vi "SLL DE AO Continous Engine.vi"(8 "error in (no error)":errorcluster) -> (0 "error out":errorcluster)   [LabVIEW 2013]
doc: "Copyright © 2005, Soliton Technologies.\nAll rights reserved."
uses:
  Controls/SLL DE DAQ Engine Options.ctl
  Controls/SLL DE AO Command LV2Global Options.ctl
  Controls/SLL DE AO Response LV2Global Options.ctl
  Controls/SLL DE AO Global Options.ctl
  Controls/SLL DE AO Circular Buffer Options.ctl
  Controls/SLL DE AO Min Max Range Checking Options.ctl
  Controls/SLL DE DAQ Global Options.ctl
  Controls/SLL DE DAQ Global Elements.ctl
  Controls/SLL DE DAQ Engine Channel Types.ctl
  Controls/SLL DE DAQ Parameters LV2Global Options.ctl
  Controls/SLL DE AO Safe Value Global Options.ctl
  <vilib>/DAQmx/configure/timing.llb/DAQmx Timing (Sample Clock).vi
  <vilib>/DAQmx/write.llb/DAQmx Write (Analog DBL 1Chan 1Samp).vi
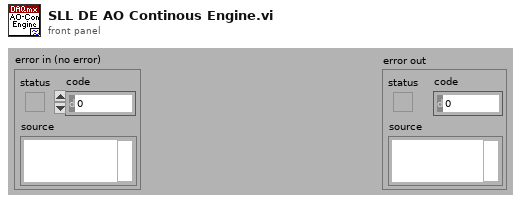
[diagram p1: front panel]
types:
  T1 = typedef "SLL DE AO Circular Buffer Options.ctl" = enum16{"Initialize", "Write 1", "Write N", "Read 1", "Read N", "Clear Data"}
  T2 = typedef "SLL DE AO Global Options.ctl" = enum16{"Init", "Write Line", "Write Array", "Read Line", "Read Array", "Read Full Status", "Restart AO", "Send to Safe Mode", "Stop AO"}
  T3 = typedef "SLL DE AO Response LV2Global Options.ctl" = enum16{"Initialize", "Send Response", "Check Response", "Close"}
  T4 = typedef "SLL DE AO Command LV2Global Options.ctl" = enum16{"Init/Register Events", "Get Event Refnum", "Fire Event", "Distroy Event"}
  T5 = typedef "SLL DE DAQ Engine Options.ctl" = enum16{">Init", ">Safe Mode", ">Poll", ">Error", ">Exit", ">Restart", ">DI", ">DO", ">AI", ">AO", ">Start Task", ">Stop Task"}
  T6 = typedef "SLL DE DAQ Parameters LV2Global Options.ctl" = enum16{"Read", "Write"}
  T7 = typedef "SLL DE DAQ Engine Channel Types.ctl" = enum16{"Analog Input", "Analog Output", "Digital Input", "Digital Output"}
  T8 = typedef "SLL DE DAQ Global Elements.ctl" = enum16{"AI Error", "AO Error", "DI Error", "DO Error", "AI Restart", "DI Restart", "AI Running", "AO Running", "DI Running", "DO Running", "DAQ Exit?"}
  T9 = typedef "SLL DE DAQ Global Options.ctl" = enum16{"Init", "Write 1", "Read 1", "Write Array", "Read Array", "Clear"}
  T10 = typedef "SLL DE AO Min Max Range Checking Options.ctl" = enum16{"Initalize Channel Range", "Check Single AO Channel", "Check Multiple AO Channels"}
  T11 = typedef "SLL DE AO Safe Value Global Options.ctl" = enum16{"Read", "Write"}
  T12 = cluster{"Previous AO Data":dbl[], "Array of AO Task":refnum<k21>[], "Execute For":string, "Channel Order":i32[], "AO Sampling Rate (Samples/Sec)":dbl}
  T13 = typedef "SLL DE DAQ Engine Parameters.ctl" = cluster{"Enable Engines":cluster{"AI Enable":bool, "AO Enable":bool, "DI Enable":bool, "DO Enable":bool}, "DAQ Control Type":cluster{"Analog Input":enum16{"Finite", "Continuous", "Driver"}, "Analog Output":enum16{"Finite", "Continuous", "Driver"}, "Digital Input":enum16{"Finite", "Continuous", "Driver"}, "Digital Output":enum16{"Finite", "Continuous", "Driver"}}, "DAQ Parameters":cluster{"AI Sampling Rate (Samples/Sec)":dbl, "MvgAVG Window Size (# of Points)":i32, "Enable Filter":bool, "Enable MvgAVG":bool, "Circular Buffer Size (Sec)":dbl, "AO Sampling Rate (Samples/Sec)":dbl, "Graph Update Rate (Samples/Sec)":dbl, "File Logging Rate (Samples/Sec)":i32}, "AO Safe Values":cluster{"Analog Outputs Name":T14, "Analog Outputs Safe Value":dbl}[], "DO Safe Values":cluster{"Digital Outputs Name":T15, "Digital Outputs Safe Value":bool}[], "DO Interconnected Lines":cluster{"First DO Line":string, "Second DO Line":string}[], "AI Channels Unit":cluster{"Channel Name":T16, "Channel Type":T17}[], "Units Information":cluster{"Channel Type":T17, "Unit Text":string, "Maximum":dbl, "Minmum":dbl, "Increments":dbl}[]}
  T14 = typedef "SLL DE List of Analog Outputs.ctl" = enum16{"None"}
  T15 = typedef "SLL DE List of Digital Outputs.ctl" = enum16{"STATION1_START TEST", "STATION1_STOP TEST", "STATION1_LIGHT1", "STATION1_LIGHT2", "STATION1_LIGHT3", "STATION1_SELECT_TEST", "STATION2_START TEST", "STATION2_STOP TEST", "STATION2_LIGHT1", "STATION2_LIGHT2", "STATION2_LIGHT3", "STATION2_SELECT_TEST", "STATION3_START TEST", "STATION3_STOP TEST", "STATION3_LIGHT1", "STATION3_LIGHT2", "STATION3_LIGHT3", "STATION3_SELECT_TEST", "STATION4_START TEST", "STATION4_STOP TEST", "STATION4_LIGHT1", "STATION4_LIGHT2", "STATION4_LIGHT3", "STATION4_SELECT_TEST"}
  T16 = typedef "SLL DE List of Analog Inputs.ctl" = enum16{"None"}
  T17 = typedef "SLL DE List of AI Channel Type.ctl" = enum16{"Pressure", "Flow", "Temperature", "Time Scale", "Voltage", "Current", "Frequency", "Sound", "Speed", "Torque", "Distance", "Channel Type 1", "Channel Type 2", "Channel Type 3"}
  T18 = enum16{"Left Button", "Center Button", "Right Button", "Window Close"}
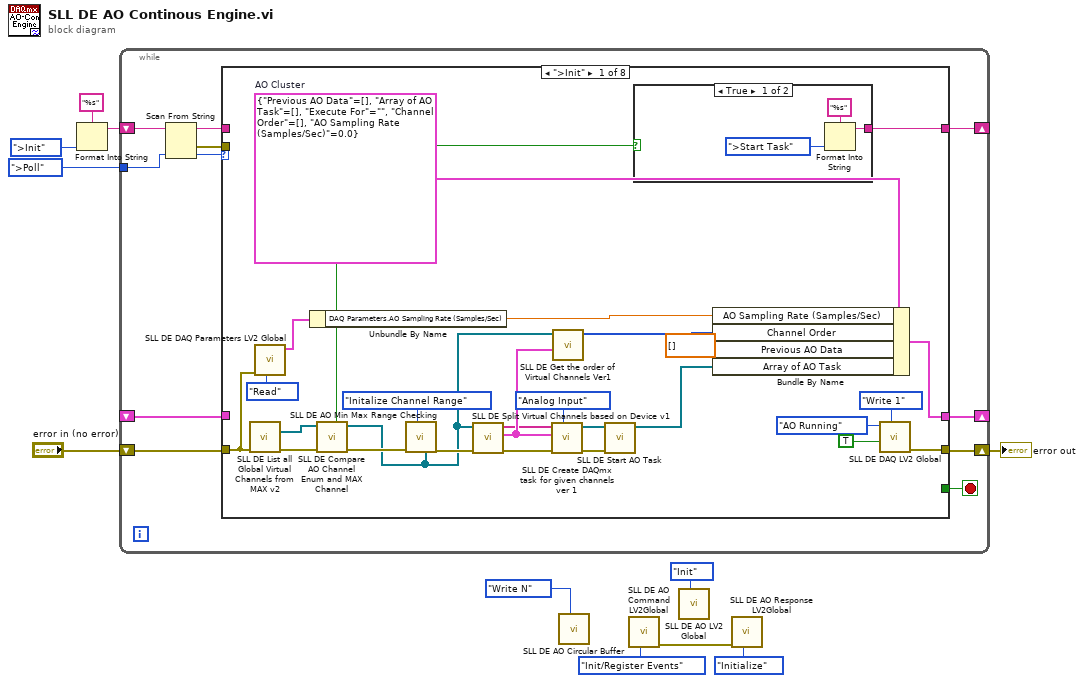
[diagram p0: block diagram]
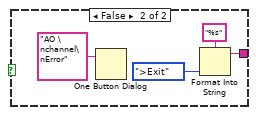
[diagram p2: hidden frame]
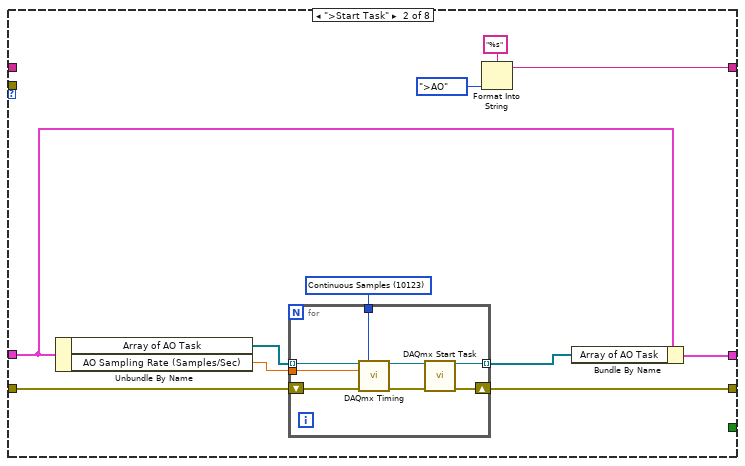
[diagram p3: hidden frame]
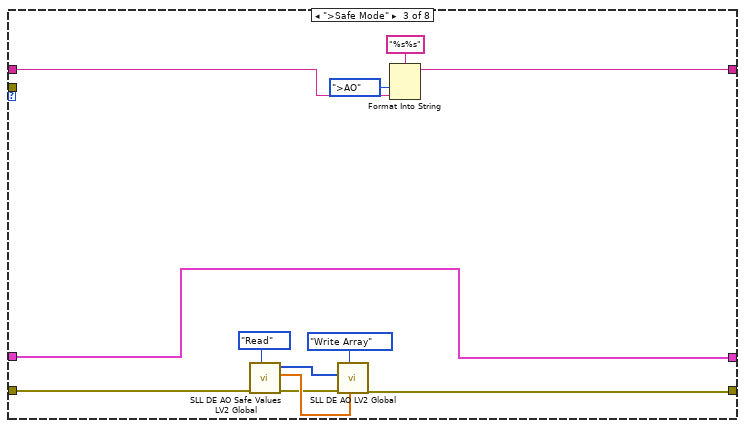
[diagram p4: hidden frame]
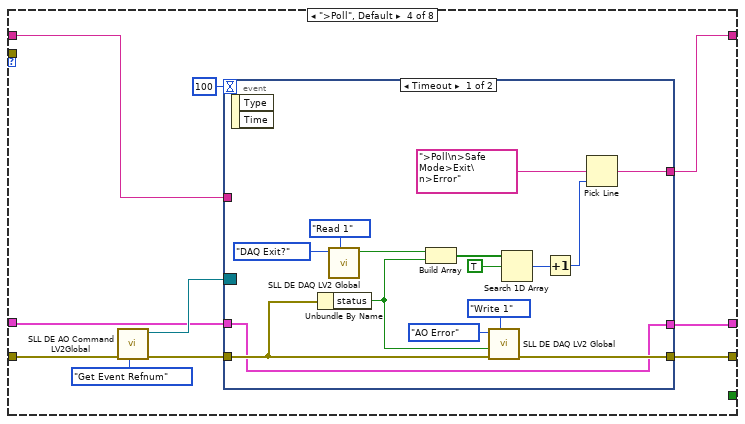
[diagram p5: hidden frame]
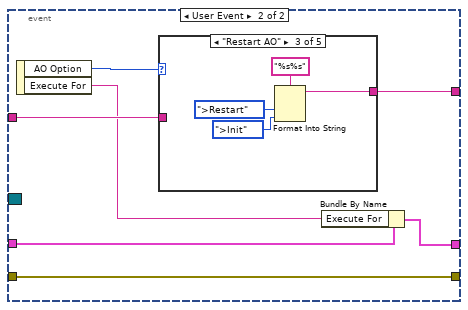
[diagram p6: hidden frame]
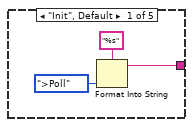
[diagram p7: hidden frame]
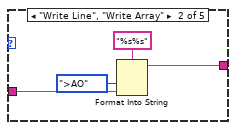
[diagram p8: hidden frame]
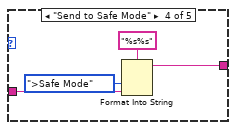
[diagram p9: hidden frame]
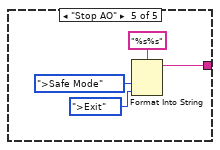
[diagram p10: hidden frame]
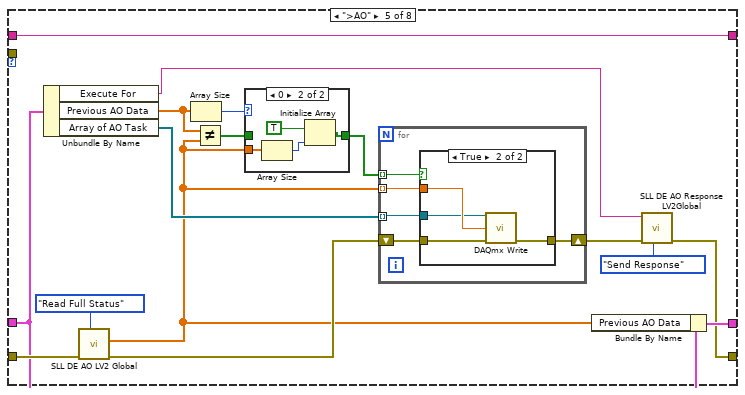
[diagram p11: hidden frame]
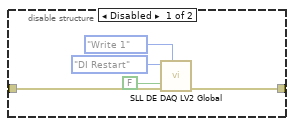
[diagram p15: hidden frame]
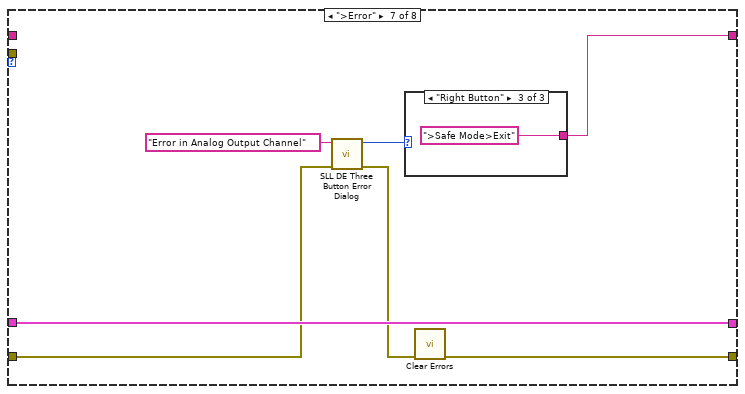
[diagram p16: hidden frame]
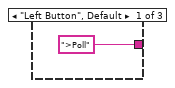
[diagram p17: hidden frame]
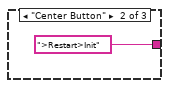
[diagram p18: hidden frame]
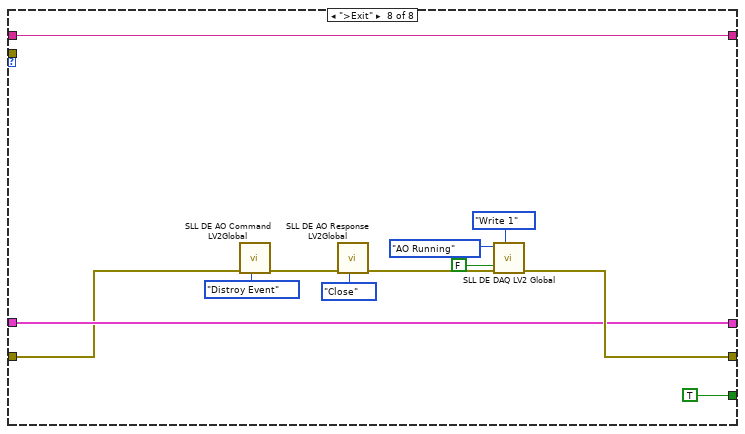
[diagram p19: hidden frame]
diagram:
  n1 = Format Into String(format string="%s", SLL_DE_DAQ_Engine_Options.">Init" ("DAQ Options")) -> (resulting string=w7:string)  [unwired: 2 in, 1 out]
  n2 = while {
    shift-right: [w21] -> w10
    shift-left: "error in (no error)" -> [w22]
    shift-right: [w20] -> _
    shift-left: _ -> [w19]
    shift-right: [w15] -> _
    shift-left: w7 -> [w18]
    tunnel: SLL_DE_DAQ_Engine_Options.">Poll" ("DAQ Options") -> [w12]
    stop <- w14 stop-if-true
    n3 = Scan From String(input string=w18, default 1=w12) -> (remaining string=w17:string, error out=w16:errorcluster, output 1=w13:T5)  [unwired: 3 in, 1 out]
    n4 = case shown="\">Init\"" w13 {
      tunnel: w22 -> [w29 w61 w83 w97 w153 w171 w184 w194]
      tunnel: [w34 w60 w76 w96 w141 w170 w183 w196] -> w21
      tunnel: [w48 w57 w81 w88 w151 w172 w186 w195] -> w20
      tunnel: w19 -> [_ w58 w81 w89 w152 w172 w186 w195]
      tunnel: w17 -> [_ _ w80 w94 w154 w173 _ w201]
      tunnel: w16 -> [_ _ _ _ _ _ _ _]
      tunnel: [w49 w64 w79 w95 w154 w173 w181 w201] -> w15
      tunnel: [_ _ _ _ _ _ _ TRUE] -> w14
      frame ">Init" {
        w40 = T12 {"Previous AO Data"=[], "Array of AO Task"=[], "Execute For"="", "Channel Order"=[], "AO Sampling Rate (Samples/Sec)"=0.0}  # AO Cluster
        n5 = call "SLL DE List all Global Virtual Channels from MAX v2.vi"("error in (no error)"=w29) -> ("error out"=w47:errorcluster, "Analog Output"=w39:refnum<k21>[])  [unwired: 4 in, 5 out]
        n6 = call "SLL DE DAQ Parameters LV2 Global.vi"("Option"=SLL_DE_DAQ_Parameters_LV2Global_Options."Read", "Error in (no error)"=w29) -> ("Global Info"=w30:T13)  [unwired: 8 in, 1 out]
        n7 = Unbundle By Name(w30) -> ("DAQ Parameters.AO Sampling Rate (Samples/Sec)"=w28:dbl)
        n8 = call "SLL DE Compare AO Channel Enum and MAX Channel.vi"("error in (no error)"=w47, "Analog Output Channels"=w39) -> ("error out"=w44:errorcluster, "Channels Out"=w26:refnum<k21>[], "Pass?"=w46:bool)  [unwired: 7 in]
        n9 = call "SLL DE AO Min Max Range Checking.vi"("Analog Output Channels"=w26, "Option"=SLL_DE_AO_Min_Max_Range_Checking_Options."Initalize Channel Range", "error in (no error)"=w44) -> ("error out"=w33:errorcluster)  [unwired: 6 in, 2 out]
        n10 = call "SLL DE Split Virtual Channels based on Device v1.vi"("error in (no error)"=w33, "GlobalChans"=w26) -> ("error out"=w36:errorcluster, "Channel Array"=w35:cluster{"Device Channel List":string[]}[], "Devices Names"=w27:string[])  [unwired: 7 in]
        n11 = call "SLL DE Create DAQmx task for given channels ver 1.vi"("Channel Type"=SLL_DE_DAQ_Engine_Channel_Types."Analog Input", "error in (no error)"=w36, "Channel Array"=w35, "Devices Names"=w27) -> ("error out"=w25:errorcluster, "Array of Tasks"=w24:refnum<k21>[])  [unwired: 6 in]
        n12 = call "SLL DE Get the order of Virtual Channels Ver1.vi"("Channel Array"=w35, "Virtial Channels Info"=w26) -> ("Channel Order"=w32:i32[])  [unwired: 8 in, 1 out]
        n13 = call "SLL DE Start AO Task.vi"("error in (no error)"=w25, "Array of AO Task"=w24) -> ("Array of AO Task Out"=w23:refnum<k21>[])  [unwired: 8 in, 1 out]
        n14 = case shown="True" w46 {
          tunnel: [w50 w53] -> w49
          frame True {
            n15 = Format Into String(format string="%s", SLL_DE_DAQ_Engine_Options.">Start Task" ("DAQ Options")) -> (resulting string=w50:string)  [unwired: 2 in, 1 out]
          }
          frame False {
            n16 = One Button Dialog(message="AO \nchannel\nError") -> ()  [unwired: 1 in, 1 out]
            n17 = Format Into String(format string="%s", SLL_DE_DAQ_Engine_Options.">Exit" ("DAQ Options")) -> (resulting string=w53:string)  [unwired: 2 in, 1 out]
          }
        }
        n18 = Bundle By Name(cluster=w40, "AO Sampling Rate (Samples/Sec)"=w28, "Channel Order"=w32, "Previous AO Data"=dbl[] [], "Array of AO Task"=w23) -> (w48:T12)
        n19 = call "SLL DE DAQ LV2 Global.vi"("Option"=SLL_DE_DAQ_Global_Options."Write 1", "Status In"=TRUE, "Element"=SLL_DE_DAQ_Global_Elements."AO Running") -> ("error out"=w34:errorcluster)  [unwired: 6 in, 2 out]
      }
      frame ">Start Task" {
        w67 = 10123 items=["Finite Samples"=10178, "Continuous Samples"=10123, "Hardware Timed Single Point"=12522] ("sample mode")
        n20 = Unbundle By Name(w58) -> ("Array of AO Task"=w63:refnum<k21>[], "AO Sampling Rate (Samples/Sec)"=w62:dbl)
        n21 = for {
          tunnel: w67 -> [w72]
          tunnel: w62 -> [w71]
          shift-right: [w73] -> w60
          shift-left: w61 -> [w75]
          tunnel: w63 -> [w69] mode=indexing
          tunnel: [w68] -> w59 mode=indexing
          n22 = call-poly <vilib>:"DAQmx Timing.vi"("task/channels in"=w69, "sample mode"=w72, "rate"=w71, "error in"=w75) -> ("task out"=w70:refnum<k21>, "error out"=w74:errorcluster)  [unwired: 3 in, 7 out]
          n23 = call <vilib>:"DAQmx Start Task.vi"("task/channels in"=w70, "error in"=w74) -> ("task out"=w68:refnum<k21>, "error out"=w73:errorcluster)  [unwired: 12 out]
        }
        n24 = Format Into String(format string="%s", SLL_DE_DAQ_Engine_Options.">AO" ("DAQ Options")) -> (resulting string=w64:string)  [unwired: 2 in, 1 out]
        n25 = Bundle By Name(cluster=w58, "Array of AO Task"=w59) -> (w57:T12)
      }
      frame ">Safe Mode" {
        n26 = call "SLL DE AO Safe Values LV2 Global.vi"("Cases"=SLL_DE_AO_Safe_Value_Global_Options."Read", "error in (no error)"=w83) -> ("error out"=w84:errorcluster, "Value Array Out"=w85:dbl[], "Elements Out"=w86:T14[])  [unwired: 7 in]
        n27 = call "SLL DE AO LV2 Global.vi"("AO value Array"=w85, "AO Option"=SLL_DE_AO_Global_Options."Write Array", "error in (no error)"=w84, "AO Channel Name Array"=w86) -> ("error out"=w76:errorcluster)  [unwired: 4 in, 3 out]
        n28 = Format Into String(format string="%s%s", SLL_DE_DAQ_Engine_Options.">AO" ("DAQ Options"), w80) -> (resulting string=w79:string)  [unwired: 2 in, 1 out]
      }
      frame ">Poll", Default {
        n29 = call "SLL DE AO Command LV2Global.vi"("Option"=SLL_DE_AO_Command_LV2Global_Options."Get Event Refnum", "Error in (no error)"=w97) -> ("Error out"=w93:errorcluster, "Event Registration Refnum"=w92:refnum<event-registration>)  [unwired: 8 in]
        n30 = event shown="[0] Timeout" {
          selector: w92 -> [_ _]
          dyn-events: _ -> [_ _]
          timeout: 100 -> [_ _]
          tunnel: w93 -> [w103 w118]
          tunnel: [w104 w118] -> w96
          tunnel: [w102 w116] -> w95
          tunnel: w94 -> [_ w117]
          tunnel: w89 -> [w101 w115]
          tunnel: [w101 w113] -> w88
          event Timeout {
            n31 = event-data() -> ()  [unwired: 1 in, 2 out]
            n32 = Unbundle By Name(w103) -> ("status"=w112:bool)
            n33 = call "SLL DE DAQ LV2 Global.vi"("Option"=SLL_DE_DAQ_Global_Options."Read 1", "Element"=SLL_DE_DAQ_Global_Elements."DAQ Exit?") -> ("Status Out"=w98:bool)  [unwired: 7 in, 2 out]
            n34 = Build Array(w98, w112) -> (w106:bool[])
            n35 = call "SLL DE DAQ LV2 Global.vi"("Option"=SLL_DE_DAQ_Global_Options."Write 1", "error in (no error)"=w103, "Status In"=w112, "Element"=SLL_DE_DAQ_Global_Elements."AO Error") -> ("error out"=w104:errorcluster)  [unwired: 5 in, 2 out]
            n36 = Search 1D Array(1D array=w106, element=TRUE) -> (index of element=w108:i32)  [unwired: 1 in]
            n37 = Increment(x=w108) -> (x+1=w109:i32)
            n38 = Pick Line(multi-line string=">Poll\n>Safe Mode>Exit\n>Error", line index=w109) -> (output string=w102:string)  [unwired: 1 in]
          }
          event User Event {
            n39 = event-data() -> ("AO Option"=w119:T2, "Execute For"=w114:string)  [unwired: 1 in]
            n40 = case shown="\"Restart AO\"" w119 {
              tunnel: w117 -> [_ w124 _ w132 _]
              tunnel: [w120 w123 w127 w131 w136] -> w116
              frame "Init", Default {
                n41 = Format Into String(format string="%s", SLL_DE_DAQ_Engine_Options.">Poll" ("DAQ Options")) -> (resulting string=w120:string)  [unwired: 2 in, 1 out]
              }
              frame "Write Line", "Write Array" {
                n42 = Format Into String(format string="%s%s", SLL_DE_DAQ_Engine_Options.">AO" ("DAQ Options"), w124) -> (resulting string=w123:string)  [unwired: 2 in, 1 out]
              }
              frame "Restart AO" {
                n43 = Format Into String(format string="%s%s", SLL_DE_DAQ_Engine_Options.">Restart" ("DAQ Options"), SLL_DE_DAQ_Engine_Options.">Init" ("DAQ Options")) -> (resulting string=w127:string)  [unwired: 2 in, 1 out]
              }
              frame "Send to Safe Mode" {
                n44 = Format Into String(format string="%s%s", SLL_DE_DAQ_Engine_Options.">Safe Mode" ("DAQ Options"), w132) -> (resulting string=w131:string)  [unwired: 2 in, 1 out]
              }
              frame "Stop AO" {
                n45 = Format Into String(format string="%s%s", SLL_DE_DAQ_Engine_Options.">Safe Mode" ("DAQ Options"), SLL_DE_DAQ_Engine_Options.">Exit" ("DAQ Options")) -> (resulting string=w136:string)  [unwired: 2 in, 1 out]
              }
            }
            n46 = Bundle By Name(cluster=w115, "Execute For"=w114) -> (w113:T12)
          }
        }
      }
      frame ">AO" {
        n47 = Unbundle By Name(w152) -> ("Execute For"=w140:string, "Previous AO Data"=w147:dbl[], "Array of AO Task"=w149:refnum<k21>[])
        n48 = call "SLL DE AO LV2 Global.vi"("AO Option"=SLL_DE_AO_Global_Options."Read Full Status", "error in (no error)"=w153) -> ("error out"=w148:errorcluster, "Analog Output Array Value"=w143:dbl[])  [unwired: 6 in, 2 out]
        n49 = Array Size(array=w147) -> (size(s)=w146:i32)
        n50 = Not Equal?(x=w147, y=w143) -> (x != y?=w145:bool[])
        n51 = case shown="0" w146 {
          tunnel: w145 -> [w155 _]
          tunnel: [w155 w158] -> w144
          tunnel: w143 -> [_ w157]
          frame Default {
          }
          frame 0 {
            n52 = Array Size(array=w157) -> (size(s)=w156:i32)
            n53 = Initialize Array(TRUE, w156) -> (w158:bool[])
          }
        }
        n54 = for {
          tunnel: w144 -> [w161] mode=indexing
          tunnel: w143 -> [w164] mode=indexing
          shift-right: [w162] -> w142
          shift-left: w148 -> [w163]
          tunnel: w149 -> [w160] mode=indexing
          n55 = case shown="True" w161 {
            tunnel: w164 -> [_ w167]
            tunnel: w163 -> [w165 w169]
            tunnel: [w165 w168] -> w162
            tunnel: w160 -> [_ w166]
            frame False {
            }
            frame True {
              n56 = call-poly <vilib>:"DAQmx Write.vi"("task/channels in"=w166, "data"=w167, "error in"=w169) -> ("error out"=w168:errorcluster)  [unwired: 10 in, 2 out]
            }
          }
        }
        n57 = Bundle By Name(cluster=w152, "Previous AO Data"=w143) -> (w151:T12)
        n58 = call "SLL DE AO Response LV2Global.vi"("Option"=SLL_DE_AO_Response_LV2Global_Options."Send Response", "Error in (no error)"=w142, "Executed For?"=w140) -> ("Error out"=w141:errorcluster)  [unwired: 7 in, 1 out]
      }
      frame ">Restart" {
        n59 = disable-structure shown="Enabled" {
          disable-tunnel: w171 -> [w175 w179]
          disable-tunnel: [w174 w179] -> w170
          frame Disabled {
            n60 = call "SLL DE DAQ LV2 Global.vi"("Option"=SLL_DE_DAQ_Global_Options."Write 1", "error in (no error)"=w175, "Status In"=FALSE, "Element"=SLL_DE_DAQ_Global_Elements."DI Restart") -> ("error out"=w174:errorcluster)  [unwired: 5 in, 2 out]
          }
          frame Enabled {
          }
        }
      }
      frame ">Error" {
        n61 = call "SLL DE Three Button Error Dialog.vi"("Error In"=w184, "Window Title"="Error in Analog Output Channel") -> ("Error Out"=w180:errorcluster, "Which Button?"=w182:T18)  [unwired: 8 in]
        n62 = case shown="\"Right Button\"" w182 {
          tunnel: [">Poll" ("Window Title") ">Restart>Init" ("Window Title") ">Safe Mode>Exit" ("Window Title")] -> w181
          frame "Left Button", Default {
          }
          frame "Center Button" {
          }
          frame "Right Button" {
          }
        }
        n63 = call <vilib>:"Clear Errors.vi"("error in (no error)"=w180) -> ("error out"=w183:errorcluster)  [unwired: 6 in]
      }
      frame ">Exit" {
        n64 = call "SLL DE AO Command LV2Global.vi"("Option"=SLL_DE_AO_Command_LV2Global_Options."Distroy Event", "Error in (no error)"=w194) -> ("Error out"=w191:errorcluster)  [unwired: 8 in, 1 out]
        n65 = call "SLL DE AO Response LV2Global.vi"("Option"=SLL_DE_AO_Response_LV2Global_Options."Close", "Error in (no error)"=w191) -> ("Error out"=w190:errorcluster)  [unwired: 8 in, 1 out]
        n66 = call "SLL DE DAQ LV2 Global.vi"("Option"=SLL_DE_DAQ_Global_Options."Write 1", "error in (no error)"=w190, "Status In"=FALSE, "Element"=SLL_DE_DAQ_Global_Elements."AO Running") -> ("error out"=w196:errorcluster)  [unwired: 5 in, 2 out]
      }
    }
  }
  "error out" <- w10
  n67 = call "SLL DE AO Circular Buffer.vi"("Options"=SLL_DE_AO_Circular_Buffer_Options."Write N") -> ()  [unwired: 7 in, 4 out]
  n68 = call "SLL DE AO Command LV2Global.vi"("Option"=SLL_DE_AO_Command_LV2Global_Options."Init/Register Events") -> ("Error out"=w4:errorcluster)  [unwired: 9 in, 1 out]
  n69 = call "SLL DE AO LV2 Global.vi"("AO Option"=SLL_DE_AO_Global_Options."Init") -> ()  [unwired: 7 in, 4 out]
  n70 = call "SLL DE AO Response LV2Global.vi"("Option"=SLL_DE_AO_Response_LV2Global_Options."Initialize", "Error in (no error)"=w4) -> ()  [unwired: 8 in, 2 out]
